vi "DHE_SendAsync.vi"(7 "type":enum16{"ERROR", "WARNING", "INFO", "CHANGED"}(ring)=enum."INFO", 9 "Message":string) -> ()   [LabVIEW 2016]
uses:
  DBSHAND/private/vis/DatabaseHand_Element_Get(string).vi
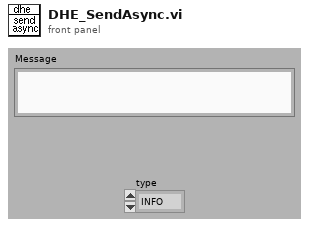
[diagram p1: front panel]
types:
  T1 = typedef "DatabaseHand_RefNum.ctl" = refnum<vi>
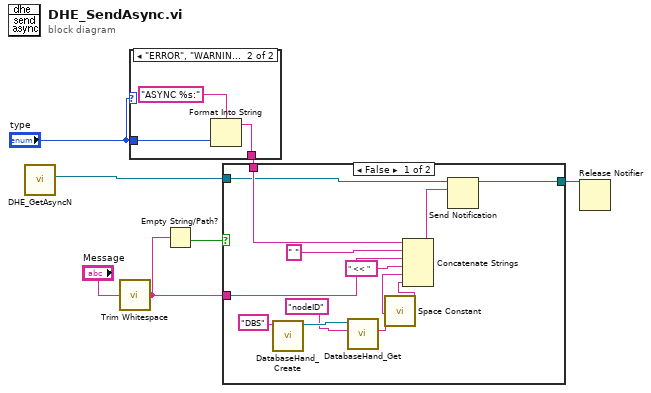
[diagram p0: block diagram]
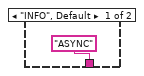
[diagram p3: hidden frame]
diagram:
  n1 = call "DHE_GetAsyncN.vi"() -> ("asyncN"=w6:refnum<notifier>)  [unwired: 11 out]
  n2 = call <vilib>:"Trim Whitespace.vi"("string"="Message") -> ("trimmed string"=w3:string)  [unwired: 1 in]
  n3 = case shown="\"ERROR\", \"WARNING\", \"CHANGED\"" "type" {
    tunnel: "type" -> [_ w11]
    tunnel: ["ASYNC" w9] -> w7
    frame "INFO", Default {
    }
    frame "ERROR", "WARNING", "CHANGED" {
      n4 = Format Into String(format string="ASYNC %s:", w11) -> (resulting string=w9:string)  [unwired: 2 in, 1 out]
    }
  }
  n5 = Empty String/Path?(string/path=w3) -> (empty?=w2:bool)
  n6 = case shown="False" w2 {
    tunnel: w7 -> [w22 _]
    tunnel: w3 -> [w20 _]
    tunnel: w6 -> [w19 w24]
    tunnel: [w12 w24] -> w1
    frame False {
      n7 = call "DatabaseHand_Create.vi"("Name"="DBS") -> ("Database RefNum out"=w17:T1)  [unwired: 1 in, 9 out]
      n8 = call-poly "DatabaseHand_Get.vi"("name"="nodeID", "Database RefNum in"=w17) -> ("value"=w14:string)  [unwired: 3 in, 6 out]
      n9 = call <vilib>:"Space Constant.vi"() -> ("String"=w13:string)
      n10 = Concatenate Strings(w22, " " ("string"), w20, " << " ("string"), w14, w13) -> (w23:string)
      n11 = Send Notification(notification=w23, notifier=w19) -> (notifier out=w12:refnum<notifier>)  [unwired: 1 in, 1 out]
    }
    frame True {
    }
  }
  n12 = Release Notifier(notifier=w1) -> ()  [unwired: 1 in, 4 out]
